vi "fields.vi"(7 "httpRequestID":u32) -> ()   [LabVIEW 2011]
doc: "This VI is a state machine that can be ran from a Browser."
uses:
  server/database/Users/User Record.ctl
  <vilib>/wsapi/NI_WebServices.lvlib
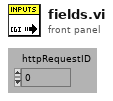
[diagram p1: front panel]
types:
  T1 = typedef "User Record.ctl" = cluster{"ixUser":i32, "sxUsername":string, "sLastName":string, "sFirstName":string, "sEmail":string, "sPassword":string, "tLoginTime":timestamp, "sLoginComputer":string, "fAdministrator":bool, "fRunSequences":bool, "fModifySequences":bool, "fRunScenarios":bool, "fModifyScenarios":bool, "fModifyTemplates":bool, "fModifyUsers":bool, "fModifyStations":bool, "fModifyFields":bool}
  T2 = typedef "Connection Refnum.ctl" = cluster{"Environment Handle":i32, "Connection Handle":i32}
  T3 = typedef "Keyed Array.ctl" = cluster{"keys":string[], "values":string[]}
  T4 = typedef "Field Record.ctl" = cluster{"ixField":i32, "iSequenceOrder":i32, "sxFieldId":string, "sxSequenceId":string, "sDisplayName":string, "sValue":string, "sUnits":string, "nDataType":T5, "nNextItem":T6, "fSystem":bool, "fSystemValue":bool, "fRequired":bool, "fSetAtTest":bool, "fTestField":bool, "fDeleted":bool, "fIndexed":bool, "fFreeList":bool}
  T5 = typedef "Field DataTypes.ctl" = enum32{"text", "numeric", "list", "timestamp", "boolean"}
  T6 = typedef "Field NextItem.ctl" = enum32{"Reset", "Retain", "Auto-Increment"}
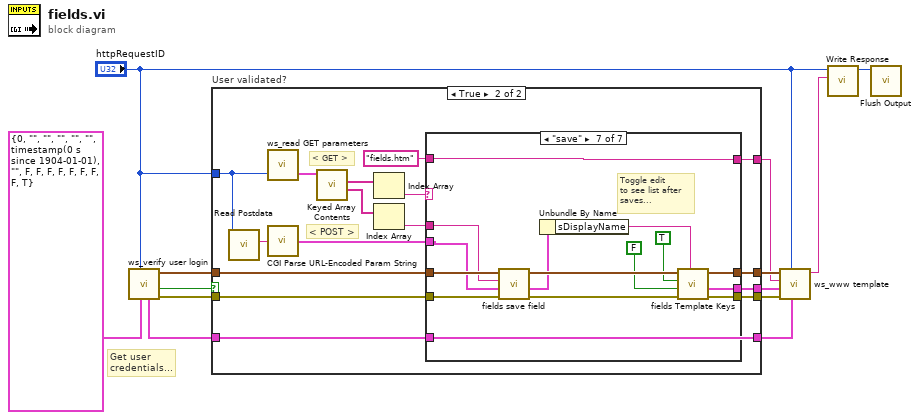
[diagram p0: block diagram]
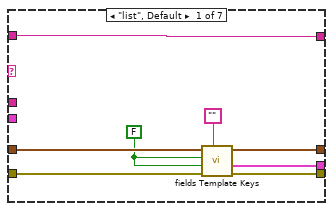
[diagram p3: hidden frame]
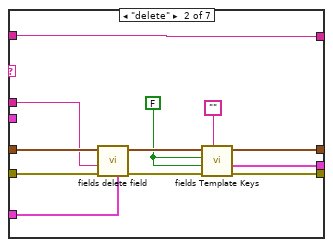
[diagram p4: hidden frame]
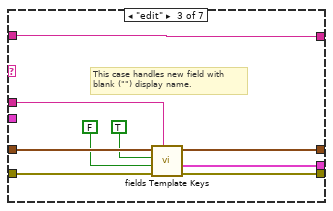
[diagram p5: hidden frame]
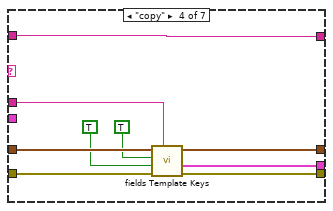
[diagram p6: hidden frame]
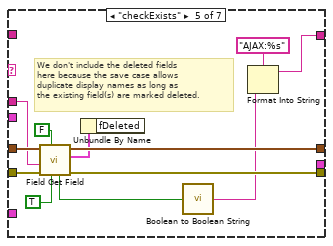
[diagram p7: hidden frame]
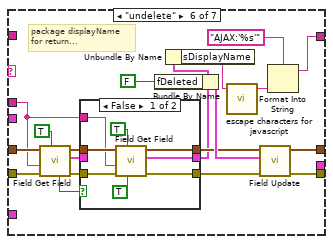
[diagram p8: hidden frame]
diagram:
  # "Get user \ncredentials..."
  n1 = call "ws_verify user login.vi"("Required Permisions"=T1 {"ixUser"=0, "sxUsername"="", "sLastName"="", "sFirstName"="", "sEmail"="", "sPassword"="", "tLoginTime"=timestamp(0 s since 1904-01-01), "sLoginComputer"="", "fAdministrator"=FALSE, "fRunSequences"=FALSE, "fModifySequences"=FALSE, "fRunScenarios"=FALSE, "fModifyScenarios"=FALSE, "fModifyTemplates"=FALSE, "fModifyUsers"=FALSE, "fModifyStations"=FALSE, "fModifyFields"=TRUE} ("User Record"), "httpRequestID"="httpRequestID") -> ("error out"=w6:errorcluster, "User Verified\nand Spartan\nAuthorized?"=w5:bool, "DB Connection Ref"=w1:T2, "User"=w4:T1)  [unwired: 6 in]
  n2 = case "User validated?" shown="True" w5 {
    tunnel: w4 -> [w14 w19]
    tunnel: w1 -> [w15 w23]
    tunnel: w6 -> [w16 w24]
    tunnel: [w16 w25] -> w13
    tunnel: [w15 w22] -> w11
    tunnel: [_ w21] -> w8
    tunnel: [_ w20] -> w9
    tunnel: [w14 w19] -> w12
    tunnel: "httpRequestID" -> [_ w18]
    frame False {
    }
    frame True {
      # "< POST >"
      # "< GET >"
      n3 = call <vilib>:"Read Postdata.vi"("httpRequestID"=w18) -> ("postdata"=w17:string)  [unwired: 8 in, 2 out]
      n4 = call "ws_read GET parameters.vi"("httpRequestID"=w18) -> ("GET query params"=w26:T3)  [unwired: 2 in]
      n5 = call <vilib>:"CGI Parse URL-Encoded Param String.vi"("url-encoded param string"=w17) -> ("params"=w27:T3)
      n6 = call <vilib>:"Keyed Array Contents.vi"("array in"=w26) -> ("values"=w30:string[], "keys"=w32:string[])  [unwired: 4 in, 1 out]
      n7 = Index Array(array=w32) -> (element=w31:string)  [unwired: 1 in]
      n8 = Index Array(array=w30) -> (element=w29:string)  [unwired: 1 in]
      n9 = case shown="\"save\"" w31 {
        tunnel: [w40 w52 w61 w70 w78 w83 w124] -> w21
        tunnel: w24 -> [w35 w47 w57 w66 w80 w100 w125]
        tunnel: [w37 w49 w58 w67 _ _ w120] -> w20
        tunnel: w29 -> [_ w43 w54 w63 w76 w88 w116]
        tunnel: [w39 w51 w60 w69 w79 w96 w121] -> w25
        tunnel: "fields.htm" ("Template (\"\")") -> [w40 w52 w61 w70 _ _ w124]
        tunnel: w23 -> [w36 w48 w56 w65 w81 w101 w126]
        tunnel: [w38 w50 w59 w68 w77 w95 w122] -> w22
        tunnel: w27 -> [_ _ _ _ _ _ w117]
        tunnel: w19 -> [_ w44 _ _ _ _ _]
        frame "list", Default {
          w33 = FALSE
          n10 = call "fields Template Keys.vi"("Display Name (\"\")"="", "error in (no error)"=w35, "Copy? (f)"=w33, "Edit? (f)"=w33, "Connection Refnum"=w36) -> ("error out"=w39:errorcluster, "Template Keys"=w37:T3, "Connection Refnum"=w38:T2)  [unwired: 1 in, 3 out]
        }
        frame "delete" {
          w41 = FALSE
          n11 = call "fields delete field.vi"("User"=w44, "error in (no error)"=w47, "Field_ID (\"\")"=w43, "Connection Refnum"=w48) -> ("error out"=w45:errorcluster, "Connection Refnum"=w46:T2)  [unwired: 6 out]
          n12 = call "fields Template Keys.vi"("Display Name (\"\")"="", "error in (no error)"=w45, "Copy? (f)"=w41, "Edit? (f)"=w41, "Connection Refnum"=w46) -> ("error out"=w51:errorcluster, "Template Keys"=w49:T3, "Connection Refnum"=w50:T2)  [unwired: 1 in, 3 out]
        }
        frame "edit" {
          # "This case handles new field with\nblank (\"\") display name."
          n13 = call "fields Template Keys.vi"("Display Name (\"\")"=w54, "error in (no error)"=w57, "Copy? (f)"=FALSE, "Edit? (f)"=TRUE, "Connection Refnum"=w56) -> ("error out"=w60:errorcluster, "Template Keys"=w58:T3, "Connection Refnum"=w59:T2)  [unwired: 1 in, 3 out]
        }
        frame "copy" {
          n14 = call "fields Template Keys.vi"("Display Name (\"\")"=w63, "error in (no error)"=w66, "Copy? (f)"=TRUE, "Edit? (f)"=TRUE, "Connection Refnum"=w65) -> ("error out"=w69:errorcluster, "Template Keys"=w67:T3, "Connection Refnum"=w68:T2)  [unwired: 1 in, 3 out]
        }
        frame "checkExists" {
          # "We don't include the deleted fields\nhere because the save case allows\nduplicate display names as long as\nthe existing field(s) are marked deleted."
          n15 = call "Field Get Field.vi"("by sDisplayName? (f, by sFieldId)"=TRUE, "Include deleted? (F)"=FALSE, "error in (no error)"=w80, "sFieldId or sDisplayName (\"\")"=w76, "Connection Refnum"=w81) -> ("error out"=w79:errorcluster, "Field"=w75:T4, "Connection Refnum"=w77:T2, "Data Present?"=w72:bool)  [unwired: 1 in, 2 out]
          n16 = Unbundle By Name(w75) -> ()  [unwired: 1 out]
          n17 = call "Boolean to Boolean String.vi"("Boolean"=w72) -> ("Boolean string"=w71:string)  [unwired: 1 in]
          n18 = Format Into String(format string="AJAX:%s", w71) -> (resulting string=w78:string)  [unwired: 2 in, 1 out]
        }
        frame "undelete" {
          # "package displayName\nfor return..."
          n19 = call "Field Get Field.vi"("Include deleted? (F)"=TRUE, "error in (no error)"=w100, "sFieldId or sDisplayName (\"\")"=w88, "Connection Refnum"=w101) -> ("error out"=w91:errorcluster, "Field"=w93:T4, "Connection Refnum"=w92:T2, "Data Present?"=w94:bool)  [unwired: 2 in, 2 out]
          n20 = case shown="False" w94 {
            tunnel: w93 -> [_ w112]
            tunnel: [w105 w112] -> w86
            tunnel: [w106 w111] -> w89
            tunnel: w92 -> [w109 w111]
            tunnel: [w107 w110] -> w90
            tunnel: w91 -> [w108 w110]
            tunnel: w88 -> [w103 _]
            frame False {
              n21 = call "Field Get Field.vi"("by sDisplayName? (f, by sFieldId)"=TRUE ("Include deleted? (F)"), "Include deleted? (F)"=TRUE, "error in (no error)"=w108, "sFieldId or sDisplayName (\"\")"=w103, "Connection Refnum"=w109) -> ("error out"=w107:errorcluster, "Field"=w105:T4, "Connection Refnum"=w106:T2)  [unwired: 1 in, 3 out]
            }
            frame True {
            }
          }
          n22 = Bundle By Name(cluster=w86, "fDeleted"=FALSE) -> (w98:T4)
          n23 = Unbundle By Name(w86) -> ("sDisplayName"=w85:string)
          n24 = call "escape characters for javascript.vi"("String (\"\")"=w85) -> ("escaped String"=w84:string)  [unwired: 4 out]
          n25 = call "Field Update.vi"("error in (no error)"=w90, "Field Record"=w98, "Connection Refnum"=w89) -> ("error out"=w96:errorcluster, "Connection Refnum"=w95:T2)  [unwired: 7 out]
          n26 = Format Into String(format string="AJAX:'%s'", w84) -> (resulting string=w83:string)  [unwired: 2 in, 1 out]
        }
        frame "save" {
          # "Toggle edit\nto see list after\nsaves..."
          n27 = call "fields save field.vi"("error in (no error)"=w125, "Post (empty)"=w117, "Field Id (\"\")"=w116, "Connection Refnum"=w126) -> ("error out"=w119:errorcluster, "Field Record"=w114:T4, "Connection Refnum"=w123:T2)  [unwired: 1 in, 4 out]
          n28 = Unbundle By Name(w114) -> ("sDisplayName"=w113:string)
          n29 = call "fields Template Keys.vi"("Display Name (\"\")"=w113, "error in (no error)"=w119, "Copy? (f)"=FALSE, "Edit? (f)"=TRUE, "Connection Refnum"=w123) -> ("error out"=w121:errorcluster, "Template Keys"=w120:T3, "Connection Refnum"=w122:T2)  [unwired: 1 in, 3 out]
        }
      }
    }
  }
  n30 = call "ws_www template.vi"("User"=w12, "httpRequestID"="httpRequestID", "error in (no error)"=w13, "Template Keys (empty)"=w9, "Template (\"\")"=w8, "DB Connection Ref"=w11) -> ("HTTP Template Content"=w10:string)  [unwired: 5 in]
  n31 = call <vilib>:"Write Response.vi"("response string"=w10, "httpRequestID"="httpRequestID") -> ("httpRequestID out"=w7:u32)  [unwired: 8 in, 1 out]
  n32 = call <vilib>:"Flush Output.vi"("httpRequestID"=w7) -> ()  [unwired: 9 in, 2 out]
